vi "LASER_GetTemp.vi"(6 "error in":errorcluster) -> (0 "error out":errorcluster, 3 "temp":dbl)   [LabVIEW 2010]
uses:
  Lumencor-DLL.dll
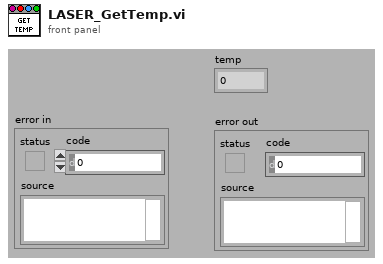
[diagram p1: front panel]
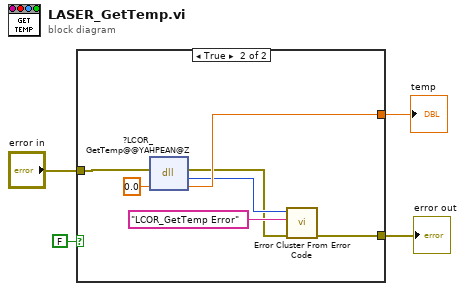
[diagram p0: block diagram]
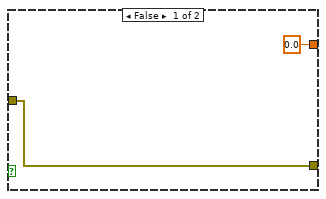
[diagram p2: hidden frame]
diagram:
  n1 = case shown="True" FALSE {
    tunnel: "error in" -> [w6 w13]
    tunnel: [0.0 ("temp") w11] -> w3
    tunnel: [w6 w7] -> w2
    frame False {
    }
    frame True {
      n2 = dll-call lib="C:/Users/tirf-user/Desktop/LabView Programs/TIRF LabView/Lumencor-DLL.dll" fn="?LCOR_GetTemp@@YAHPEAN@Z" label="LCOR_GetTemp"(error in=w13, "temp"=0.0) -> (error out=w8:errorcluster, "return type"=w9:i32, "temp"=w11:dbl)  [unwired: 2 in, 1 out]
      n3 = call <vilib>:"Error Cluster From Error Code.vi"("error in (no error)"=w8, "error message (\"\")"="LCOR_GetTemp Error" ("error message (\"\")"), "error code (0)"=w9) -> ("error out"=w7:errorcluster)  [unwired: 6 in]
    }
  }
  "temp" <- w3
  "error out" <- w2
